vi "VCS Is Recorder Triggered.vi"(8 "error in (no error)":errorcluster, 11 "axis in":cluster{"keyHandle":u32, "nodeId":u16}={"keyHandle"=0, "nodeId"=1}) -> (0 "error out":errorcluster, 1 "isTriggered":i32, 3 "axis out":cluster{"keyHandle":u32, "nodeId":u16}={"keyHandle"=0, "nodeId"=1})   [LabVIEW 2018]
doc: "<B>VCS_IsRecorderTriggered</B> returns data recorder status triggered."
uses:
  Resources/EposCmd.dll
  Resources/EposCmd64.dll
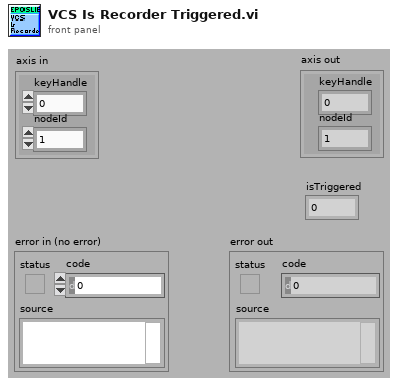
[diagram p1: front panel]
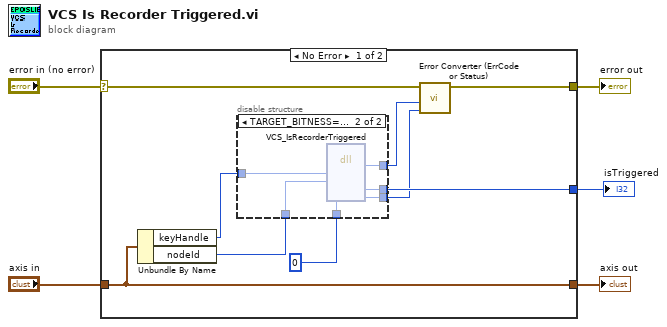
[diagram p0: block diagram]
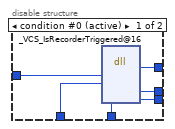
[diagram p2: hidden frame]
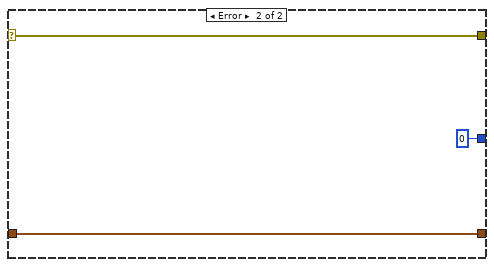
[diagram p3: hidden frame]
diagram:
  n1 = case shown="No Error" "error in (no error)" {
    selector: "error in (no error)" -> [w12 w28]
    tunnel: "axis in" -> [w14 w29]
    tunnel: [w14 w29] -> w4
    tunnel: [w13 w28] -> w3
    tunnel: [w11 0 ("pTriggered")] -> w1
    frame No Error {
      n2 = Unbundle By Name(w14) -> ("keyHandle"=w8:u32, "nodeId"=w9:u16)
      n3 = disable-structure shown="TARGET_BITNESS==64" {
        disable-tunnel: [w20 w26] -> w11
        disable-tunnel: u32 0 ("pErrorCode") -> [w19 w25]
        disable-tunnel: w9 -> [w18 w24]
        disable-tunnel: w8 -> [w17 w23]
        disable-tunnel: [w16 w22] -> w7
        disable-tunnel: [w15 w21] -> w6
        frame condition #0 (active) {
          n4 = dll-call lib="C:/Projeto em LabVIEW/EPOS-LabVIEW-Instrument-Driver-En/LabVIEW/maxon EPOS/Resources/EposCmd.*" fn="_VCS_IsRecorderTriggered@16"("KeyHandle"=w17, "NodeId"=w18, "pErrorCode"=w19) -> (w16:i32, "pTriggered"=w20:i32, "pErrorCode"=w15:u32)  [unwired: 6 in, 2 out]
        }
        frame condition #1 {
          n5 = dll-call lib="C:/setup/Resources/EposCmd64.*" fn="VCS_IsRecorderTriggered" ("EposCmd.dll:_VCS_IsRecorderTriggered@16")("KeyHandle"=w23, "NodeId"=w24, "pErrorCode"=w25) -> ("Rückgabetyp"=w22:i32, "pTriggered"=w26:i32, "pErrorCode"=w21:u32)  [unwired: 6 in, 2 out]
        }
      }
      n6 = call "Error Converter (ErrCode or Status).vi"("error code"=w6, "return type"=w7, "error in (no error)"=w12) -> ("error out"=w13:errorcluster)  [unwired: 7 in]
    }
    frame Error {
    }
  }
  "isTriggered" <- w1
  "error out" <- w3
  "axis out" <- w4
